vi "Largest Contiguous Channel Count (Transfer Group).vi"(8 "error in (no error)":errorcluster, 10 "largest contiguous channel count in (0)":u64, 11 "Transfer Group Configuration in":T1={"name"="", "direction"=enum."Tx", "cycle timing"={"priority"=0, "decimation"=1, "offset"=0}, "Transfers"=[], "settings"=[]} {"Transfers"."channels"."dst buffer offset" format="%d bytes"; "Transfers"."channels"."src buffer offset" format="%d bytes"}) -> (0 "error out":errorcluster, 2 "largest contiguous channel count out":u64, 3 "Transfer Group Configuration out":T1={"name"="", "direction"=enum."Tx", "cycle timing"={"priority"=0, "decimation"=1, "offset"=0}, "Transfers"=[], "settings"=[]} {"Transfers"."channels"."dst buffer offset" format="%d bytes"; "Transfers"."channels"."src buffer offset" format="%d bytes"})   [LabVIEW 2017, in "DSF Core.lvlib"]
uses:
  DSF Core.lvlib
  Controls/DSF Engine Transfer Group Configuration.ctl
  Controls/DSF Direction.ctl
  Controls/DSF Timing Info.ctl
  Controls/DSF Engine Transfer Configuration.ctl
  Controls/DSF Byte Order.ctl
  Controls/DSF Engine Channel Configuration.ctl
  Controls/DSF Data Type.ctl
  Controls/DSF Settings Info.ctl
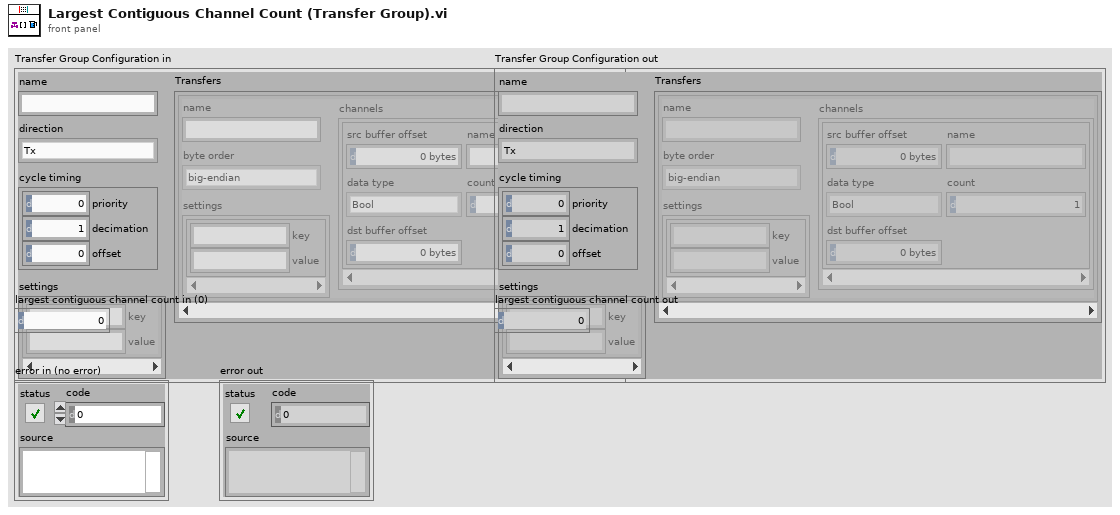
[diagram p1: front panel]
types:
  T1 = typedef "DSF Core.lvlib/DSF Engine Transfer Group Configuration.ctl" = cluster{"name":string, "direction":T2, "cycle timing":T3, "Transfers":T4[], "settings":T8}
  T2 = typedef "DSF Core.lvlib/DSF Direction.ctl" = enum8{"Tx", "Rx"}
  T3 = typedef "DSF Core.lvlib/DSF Timing Info.ctl" = cluster{"priority":u64, "decimation":u64, "offset":u64}
  T4 = typedef "DSF Core.lvlib/DSF Engine Transfer Configuration.ctl" = cluster{"name":string, "byte order":T5, "channels":T6[], "settings":T8}
  T5 = typedef "DSF Core.lvlib/DSF Byte Order.ctl" = enum8{"big-endian", "little-endian"}
  T6 = typedef "DSF Core.lvlib/DSF Engine Channel Configuration.ctl" = cluster{"src buffer offset":u64, "name":string, "data type":T7, "count":u64, "dst buffer offset":u64}
  T7 = typedef "DSF Core.lvlib/DSF Data Type.ctl" = enum8{"Bool", "SGL", "DBL", "I8", "I16", "I32", "I64", "U8", "U16", "U32", "U64"}
  T8 = typedef "DSF Core.lvlib/DSF Settings Info.ctl" = cluster{"key":string, "value":string}[]
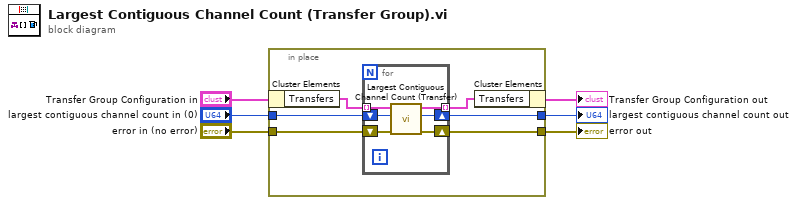
[diagram p0: block diagram]
diagram:
  n1 = in-place {
    in-place-border: "error in (no error)" -> [w12]
    in-place-border: [w11] -> w5
    in-place-border: "largest contiguous channel count in (0)" -> [w10]
    in-place-border: [w9] -> w3
    n2 = in-place-cluster #1("Transfer Group Configuration in") -> ("Transfers"=w8:T4[])
    n3 = for {
      tunnel: w8 -> [w14] mode=indexing
      tunnel: [w13] -> w7 mode=indexing
      shift-right: [w17] -> w11
      shift-left: w12 -> [w18]
      shift-right: [w15] -> w9
      shift-left: w10 -> [w16]
      n4 = call "Largest Contiguous Channel Count (Transfer).vi"("error in (no error)"=w18, "largest contiguous channel count in (0)"=w16, "Transfer Configuration in"=w14) -> ("error out"=w17:errorcluster, "largest contiguous channel count out"=w15:u64, "Transfer Configuration out"=w13:T4)  [unwired: 6 in]
    }
    n5 = in-place-cluster #1("Transfers"=w7) -> (→"Transfer Group Configuration out":T1)
  }
  "error out" <- w5
  "largest contiguous channel count out" <- w3
